vi "Read and Update Message Example.vi"(0 "GEA Inputs":T2 {"Destination" format="%.0x"; "Source" format="%.0x"}, 1 "Device Selected":i32, 2 "Retry Count":u32=5, 3 "Read Timeout (ms)":u32=500, 5 "Read Command":u8 format="%.0x", 7 "Write Command":u8 format="%.0x", 9 "Update Information":string, 11 "Error In":errorcluster, 12 "Expected Command":string=".*", 13 "Expected Data":string=".*") -> (4 "Updated Converted Data Out":T1 {"CRC" format="%04x"; "Length" format="%02x"; "Command" format="%02x"; "Destination" format="%02x"; "Source" format="%02x"}, 6 "Updated Raw Data Out":string, 15 "Error Out":errorcluster)   [LabVIEW 2014]
doc: "This VI demonstrates how to read and update data using GEA2 messages."
uses:
  type defs/Source_Destination.ctl
  type defs/Data Out.ctl
  library/GEA2_Toolkit.lvlib
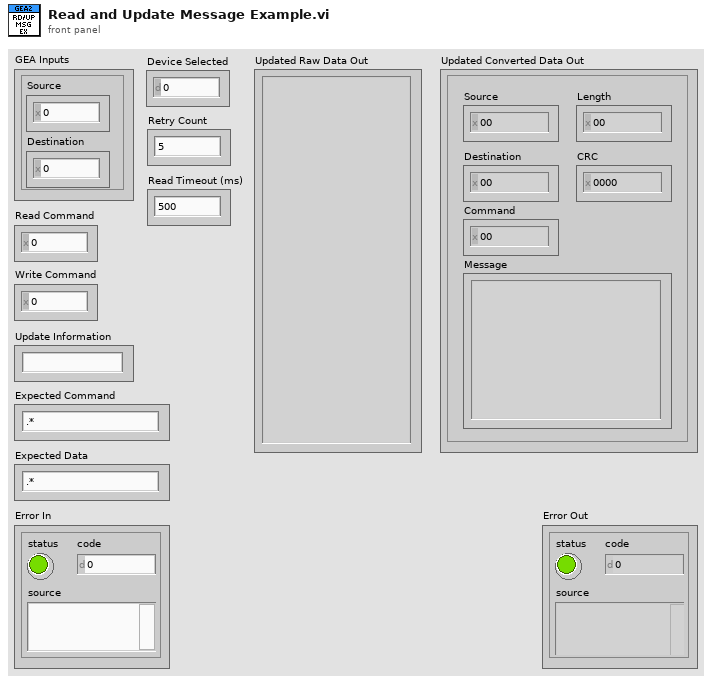
[diagram p1: front panel]
types:
  T1 = typedef "GEA2_Toolkit.lvlib/Data Out.ctl" = cluster{"Source":u8, "Destination":u8, "Command":u8, "Length":u8, "CRC":u16, "Message":string}
  T2 = typedef "GEA2_Toolkit.lvlib/Source_Destination.ctl" = cluster{"Source":u8, "Destination":u8}
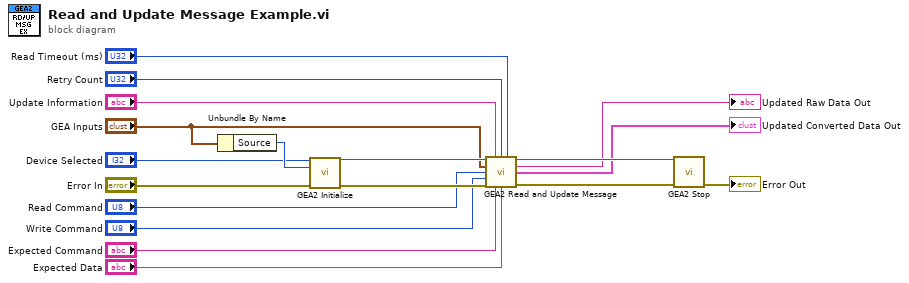
[diagram p0: block diagram]
diagram:
  n1 = Unbundle By Name("GEA Inputs") -> ("Source"=w14:u8)
  n2 = call "GEA2 Initialize.vi"("Board Index"="Device Selected", "Source Address"=w14, "error in"="Error In") -> ("GEA2 Reference Out"=w15:refnum<k24>, "error out"=w18:errorcluster)  [unwired: 10 in, 1 out]
  n3 = call "GEA2 Read and Update Message.vi"("GEA2 Reference In"=w15, "Update Information"="Update Information", "Send Retry Count"="Retry Count", "Read Timeout (ms)"="Read Timeout (ms)", "GEA Inputs"="GEA Inputs", "Read Command"="Read Command", "Write Command"="Write Command", "Error In"=w18, "Expected Command"="Expected Command", "Expected Data"="Expected Data") -> ("GEA2 Reference Out"=w16:refnum<k24>, "Updated Raw Data Out"=→"Updated Raw Data Out":string, "Updated Converted Data Out"=→"Updated Converted Data Out":T1, "Error Out"=w17:errorcluster)  [unwired: 2 in]
  n4 = call "GEA2 Stop.vi"("GEA2 Reference In"=w16, "Error In"=w17) -> ("Error Out"=→"Error Out":errorcluster)  [unwired: 13 in]
